vi "FTW-Endpoint-CreateReplier.vi"(0 "FTW Endpoint":refnum<class "FTW-Endpoint-TCP.lvclass">, 11 "error in":errorcluster) -> (4 "FTW Endpoint out":refnum<class "FTW-Endpoint-TCP.lvclass">, 15 "error out":errorcluster)   [LabVIEW 2013, in "FTW-Endpoint-TCP.lvclass"]
uses:
  FTW-Endpoint-TCP.lvclass
panel:
  # "Inputs"
  # "Outputs"
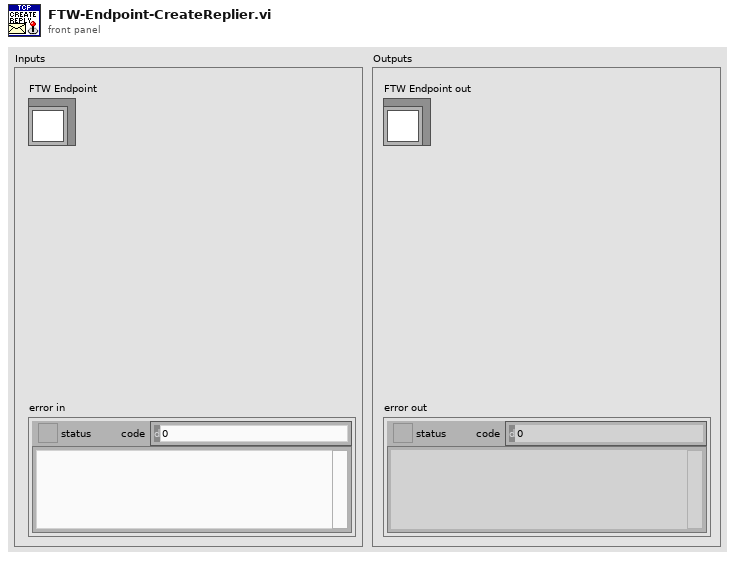
[diagram p1: front panel]
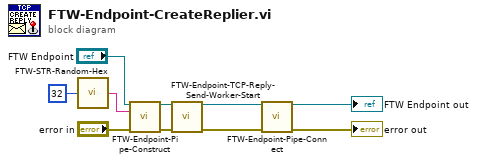
[diagram p0: block diagram]
diagram:
  n1 = call "FTW-STR-Random-Hex.vi"("String Length"=32) -> ("Random Hex String"=w4:string)  [unwired: 3 in]
  n2 = call-dynamic "FTW-Endpoint-Pipe-Construct.vi"("FTW Endpoint"="FTW Endpoint", "Address"=w4, "error in"="error in") -> ("FTW Endpoint out"=w6:refnum<class "FTW-Endpoint-TCP.lvclass">, "error out"=w7:errorcluster)  [unwired: 10 in, 1 out]
  n3 = call-dynamic "FTW-Endpoint-TCP-Reply-Send-Worker-Start.vi"("FTW-Endpoint-TCP In"=w6, "error in"=w7) -> ("FTW-Endpoint-TCP Out"=w2:refnum<class "FTW-Endpoint-TCP.lvclass">, "error out"=w8:errorcluster)  [unwired: 12 in]
  n4 = call-dynamic "FTW-Endpoint-Pipe-Connect.vi"("FTW Endpoint"=w2, "error in"=w8) -> ("FTW Endpoint out"=→"FTW Endpoint out":refnum<class "FTW-Endpoint-TCP.lvclass">, "error out"=→"error out":errorcluster)  [unwired: 12 in]
